vi "Toolkit - Alphabetize Cluster Control Target.vi"() -> ()   [LabVIEW 2018]
doc: "The target VI for the Toolkit - Cluster Control example. Do NOT modify the contents of this VI. This is needed because alphabetizing within a running VI is not possible."
panel:
  in  "Data":T1
  # "Overview: The target VI for the Toolkit - Alphabetize Cluster Control example\nInstructions:\n1. Do not modify or remove\n\nThis is needed for alphabetizing a cluster control using VI scripting and the ACE toolkit. The Front Panel will automatically be displayed when the \"Toolkit - Alphabetize Cluster Control\" example is run. The example will also automatically undo the changes and close this VI."
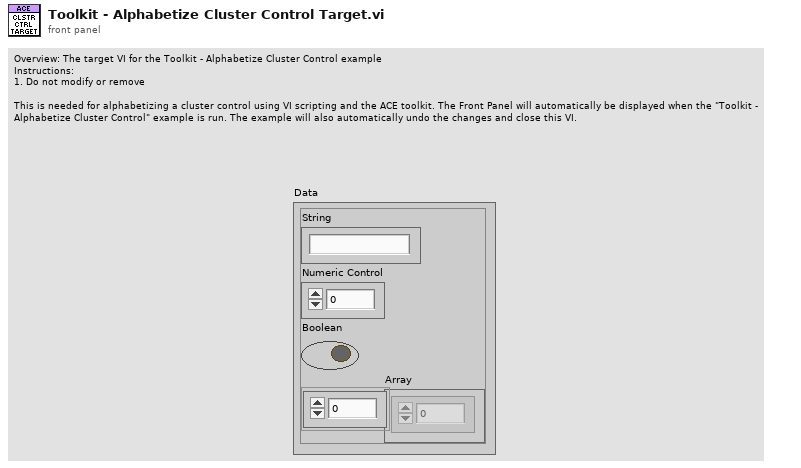
[diagram p1: front panel]
types:
  T1 = cluster{"String":string, "Numeric Control":dbl, "Boolean":bool, "Array":dbl[]}
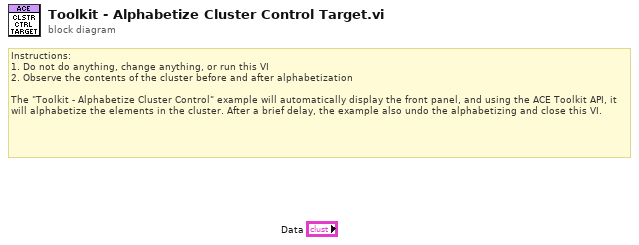
[diagram p0: block diagram]
diagram:
  # "Instructions:\n1. Do not do anything, change anything, or run this VI\n2. Observe the contents of the cluster before and after alphabetization\n\nThe \"Toolkit - Alphabetize Cluster Control\" example will automatically display the front panel, and using the ACE Toolkit API, it will alphabetize the elements in the cluster. After a brief delay, the example also undo the alphabetizing and close this VI."
